vi "FRIC_navX_Get_Displacement.vi"(7 "Update":bool) -> (2 "Displacement":T1)   [LabVIEW 2015]
doc: "This navX VI returns the velocity and displacement of the navX. This VI is only supported on firmware virsions newer than 2.2.xxx."
uses:
  TypeDefs/FRIC_navX_DecodeRegisterLengthClusterTypeDef_.ctl
  navX Library v2/_TypeDefs/Z900_navX_DeviceRegisters.ctl
  navX Library v2/navX Library v2.lvlib
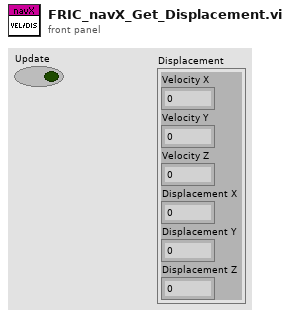
[diagram p1: front panel]
types:
  T1 = cluster{"Velocity X":dbl, "Velocity Y":dbl, "Velocity Z":dbl, "Displacement X":dbl, "Displacement Y":dbl, "Displacement Z":dbl}
  T2 = typedef "FRIC_navX_DecodeRegisterLengthClusterTypeDef_.ctl" = cluster{"Device Register":T3, "length":i32}[]
  T3 = typedef "navX Library v2.lvlib/Z900_navX_DeviceRegisters.ctl" = u8
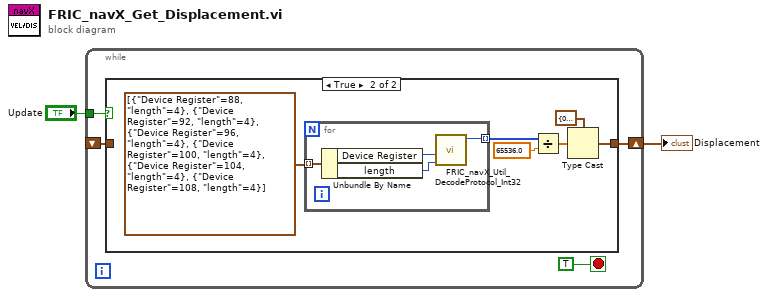
[diagram p0: block diagram]
diagram:
  n1 = while {
    shift-right: [w6] -> w2
    shift-left: _ -> [w3]
    tunnel: "Update" -> [w4]
    stop <- TRUE stop-if-true
    n2 = case shown="True" w4 {
      tunnel: [w7 w13] -> w6
      tunnel: w3 -> [w7 _]
      frame False {
      }
      frame True {
        n3 = for {
          tunnel: T2 [{"Device Register"=88, "length"=4}, {"Device Register"=92, "length"=4}, {"Device Register"=96, "length"=4}, {"Device Register"=100, "length"=4}, {"Device Register"=104, "length"=4}, {"Device Register"=108, "length"=4}] -> [w17] mode=indexing
          tunnel: [w14] -> w8 mode=indexing
          n4 = Unbundle By Name(w17) -> ("Device Register"=w16:T3, "length"=w15:i32)
          n5 = call "FRIC_navX_Util_DecodeProtocol_Int32.vi"("length"=w15, "Device Register"=w16) -> ("Value"=w14:i32)  [unwired: 8 in]
        }
        n6 = Divide(x=w8, y=65536.0) -> (x/y=w10:dbl[])
        n7 = Type Cast(type=T1 {"Velocity X"=0.0, "Velocity Y"=0.0, "Velocity Z"=0.0, "Displacement X"=0.0, "Displacement Y"=0.0, "Displacement Z"=0.0}, x=w10) -> (*(type *) &x=w13:T1)
      }
    }
  }
  "Displacement" <- w2
